vi "All Dirs to List.vi"(8 "error in (no error)":errorcluster, 11 "dir in":refnum<class "dir.lvclass">) -> (0 "error out":errorcluster, 2 "Dir List":cluster{"Name":string, "Size":i64}[](array[cluster]), 3 "dir out":refnum<class "dir.lvclass">)   [LabVIEW 2021, in "d7.lvlib" / "dir.lvclass"]
uses:
  dir.lvclass
  file/file.lvclass
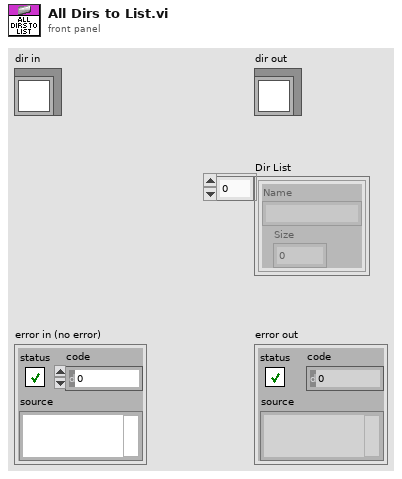
[diagram p1: front panel]
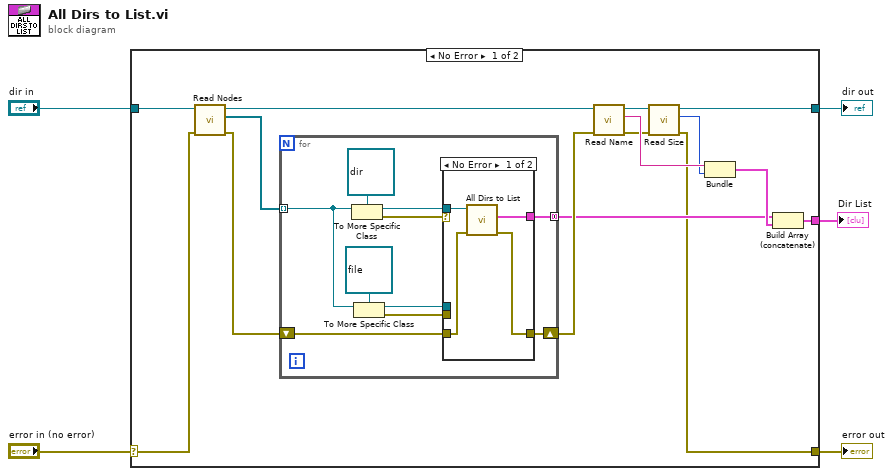
[diagram p0: block diagram]
diagram:
  n1 = case shown="No Error" "error in (no error)" {
    selector: "error in (no error)" -> [w14 w37]
    tunnel: [w6 w37] -> w4
    tunnel: [w9 w36] -> w2
    tunnel: "dir in" -> [w19 w36]
    tunnel: [w16 _] -> w1
    frame No Error {
      n2 = call-dynamic "Read Nodes.vi"("error in (no error)"=w14, "dir in"=w19) -> ("error out"=w12:errorcluster, "Nodes"=w20:refnum<class "INode.lvclass">[], "dir out"=w18:refnum<class "dir.lvclass">)  [unwired: 7 in]
      n3 = for {
        tunnel: w20 -> [w26] mode=indexing
        shift-right: [w22] -> w13
        shift-left: w12 -> [w23]
        tunnel: [w21] -> w11 mode=concatenating
        n4 = To More Specific Class(target class=refnum<class "dir.lvclass"> refnum ("d7.lvlib:dir.lvclass"), reference=w26) -> (specific class reference=w30:refnum<class "dir.lvclass">, error out=w28:errorcluster)  [unwired: 1 in]
        n5 = To More Specific Class(target class=refnum<class "file.lvclass"> refnum ("d7.lvlib:file.lvclass"), reference=w26) -> (specific class reference=w27:refnum<class "file.lvclass">, error out=w25:errorcluster)  [unwired: 1 in]
        n6 = case shown="No Error" w28 {
          tunnel: w30 -> [w34 _]
          tunnel: w27 -> [_ _]
          tunnel: w25 -> [_ _]
          tunnel: [w32 _] -> w21
          tunnel: w23 -> [w33 w35]
          tunnel: [w31 w35] -> w22
          frame No Error {
            n7 = call-dynamic "All Dirs to List.vi"("error in (no error)"=w33, "dir in"=w34) -> ("error out"=w31:errorcluster, "Dir List"=w32:cluster{"Name":string, "Size":i64}[])  [unwired: 7 in, 1 out]
          }
          frame Error {
          }
        }
      }
      n8 = call-dynamic "Read Name.vi"("error in (no error)"=w13, "node in"=w18) -> ("error out"=w7:errorcluster, "Name"=w17:string, "node out"=w10:refnum<class "dir.lvclass">)  [unwired: 7 in]
      n9 = call-dynamic "Read Size.vi"("error in (no error)"=w7, "file in"=w10) -> ("error out"=w6:errorcluster, "Size"=w8:i64, "file out"=w9:refnum<class "dir.lvclass">)  [unwired: 7 in]
      n10 = Bundle("Name"=w17, "Size"=w8) -> (w15:cluster{"Name":string, "Size":i64})  [unwired: 1 in]
      n11 = Build Array (concatenate)(w11, w15) -> (w16:cluster{"Name":string, "Size":i64}[])
    }
    frame Error {
    }
  }
  "error out" <- w4
  "dir out" <- w2
  "Dir List" <- w1
